vi "Stop Communication.vi"(8 "error in (no error)":errorcluster) -> (0 "error out":errorcluster)   [LabVIEW 2017]
uses:
  Type Definitions/Queue FG Options.ctl
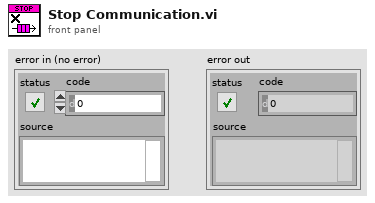
[diagram p1: front panel]
types:
  T1 = typedef "Queue FG Options.ctl" = enum16{"Set", "Get", "Read", "Write", "Destroy"}
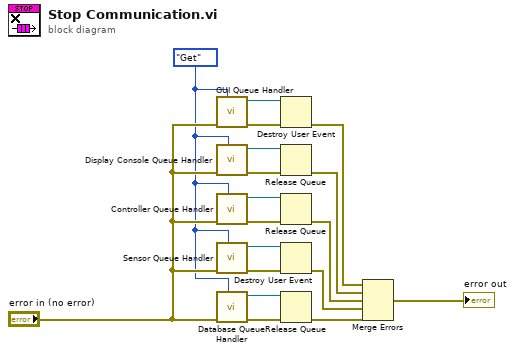
[diagram p0: block diagram]
diagram:
  w17 = Queue_FG_Options."Get" ("Action")
  n1 = call "GUI Queue Handler.vi"("Action"=w17, "error in (no error)"="error in (no error)") -> ("error out"=w15:errorcluster, "User event out"=w16:refnum<user-event>)  [unwired: 6 in, 2 out]
  n2 = call "Display Console Queue Handler.vi"("Action"=w17, "error in (no error)"="error in (no error)") -> ("error out"=w8:errorcluster, "Queue out"=w7:refnum<queue>)  [unwired: 7 in, 1 out]
  n3 = call "Controller Queue Handler.vi"("Action"=w17, "error in (no error)"="error in (no error)") -> ("error out"=w9:errorcluster, "Queue out"=w10:refnum<queue>)  [unwired: 7 in, 1 out]
  n4 = call "Sensor Queue Handler.vi"("Action"=w17, "error in (no error)"="error in (no error)") -> ("error out"=w14:errorcluster, "User event out"=w13:refnum<user-event>)  [unwired: 6 in, 2 out]
  n5 = call "Database Queue Handler.vi"("Action"=w17, "error in (no error)"="error in (no error)") -> ("error out"=w12:errorcluster, "Queue out"=w11:refnum<queue>)  [unwired: 7 in, 1 out]
  n6 = Destroy User Event(user event=w16, error in=w15) -> (error out=w5:errorcluster)
  n7 = Release Queue(queue=w7, error in (no error)=w8) -> (error out=w4:errorcluster)  [unwired: 1 in, 2 out]
  n8 = Release Queue(queue=w10, error in (no error)=w9) -> (error out=w3:errorcluster)  [unwired: 1 in, 2 out]
  n9 = Destroy User Event(user event=w13, error in=w14) -> (error out=w2:errorcluster)
  n10 = Release Queue(queue=w11, error in (no error)=w12) -> (error out=w6:errorcluster)  [unwired: 1 in, 2 out]
  n11 = Merge Errors(w5, w4, w3, w2, w6) -> (→"error out":errorcluster)
